vi "Draw_Horiz_Lines_On_Img.vi"(6 "[IN] Color":u32(colorbox)=16711680, 8 "error IN":errorcluster, 10 "[IN] Horizontal step":i32=1 min=1 max=10000 step=1, 11 "[IN] Image":T1) -> (0 "error OUT":errorcluster, 3 "[OUT] Image":T1)   [LabVIEW 2020]
uses:
  <vilib>/vision/Image Controls.llb/IMAQ Image.ctl
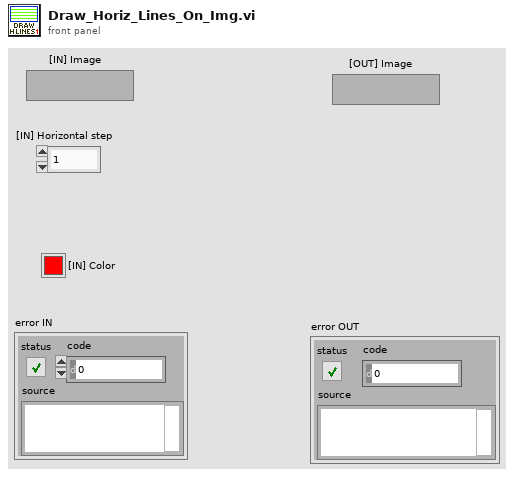
[diagram p1: front panel]
types:
  T1 = typedef "IMAQ Image.ctl" = refnum<image>
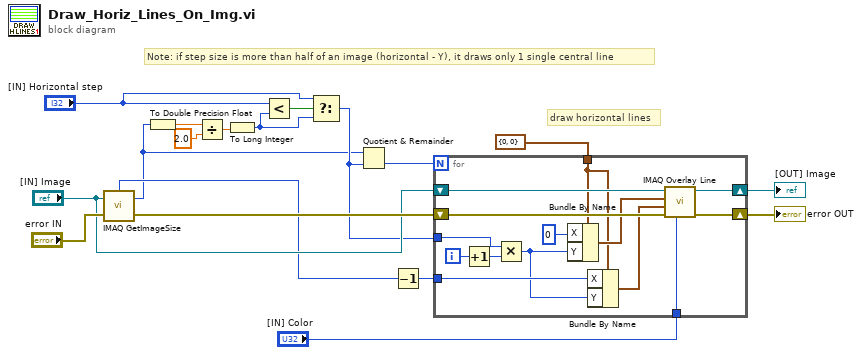
[diagram p0: block diagram]
diagram:
  # "Note: if step size is more than half of an image (horizontal - Y), it draws only 1 single central line"
  # "draw horizontal lines"
  n1 = call "IMAQ GetImageSize"("Image"="[IN] Image", "error in (no error)"="error IN") -> ("Y Resolution"=w2:i32, "X Resolution"=w3:i32, "error out"=w17:errorcluster)  [unwired: 2 in]
  n2 = To Double Precision Float(number=w2) -> (double precision float=w10:dbl)
  n3 = Divide(x=w10, y=2.0) -> (x/y=w8:dbl)
  n4 = To Long Integer(number=w8) -> (32bit integer=w5:i32)
  n5 = Less?(x="[IN] Horizontal step", y=w5) -> (x < y?=w7:bool)
  n6 = Select(t="[IN] Horizontal step", s=w7, f=w5) -> (s? t:f=w4:i32)
  n7 = Quotient & Remainder(x=w2, y=w4) -> (floor(x/y)=w1:i32)  [unwired: 1 out]
  n8 = Decrement(x=w3) -> (x-1=w14:i32)
  n9 = for {
    N: w1 -> [_]
    shift-right: [w31] -> w11
    shift-left: w17 -> [w32]
    tunnel: w4 -> [w27]
    tunnel: "[IN] Color" -> [w26]
    tunnel: w14 -> [w20]
    tunnel: cluster{"X":i32, "Y":i32} {"X"=0, "Y"=0} ("Start Point") -> [w24]
    shift-right: [w22] -> w12
    shift-left: "[IN] Image" -> [w30]
    i -> [w29]
    n10 = Increment(x=w29) -> (x+1=w28:i32)
    n11 = Multiply(x=w27, y=w28) -> (x*y=w19:i32)
    n12 = Bundle By Name(cluster=w24, "X"=0 ("Y"), "Y"=w19) -> (w25:cluster{"X":i32, "Y":i32})
    n13 = Bundle By Name(cluster=w24, "X"=w20, "Y"=w19) -> (w23:cluster{"X":i32, "Y":i32})
    n14 = call "IMAQ Overlay Line"("Color"=w26, "error in (no error)"=w32, "End Point"=w23, "Start Point"=w25, "Image"=w30) -> ("error out"=w31:errorcluster, "Image Out"=w22:T1)  [unwired: 5 in]
  }
  "[OUT] Image" <- w12
  "error OUT" <- w11
